vi "Knob Turn.vi"(0 "GEA2 Reference In":refnum<k24>, 7 "Button":T1=enum."Position 1", 11 "Error In":errorcluster) -> (4 "GEA2 Reference Out":refnum<k24>, 15 "Error Out":errorcluster)   [LabVIEW 2018, in "TL27.lvlib"]
uses:
  Projects/TL27.lvlib
  type defs/Encoder Position.ctl
  D:/Common/LabVIEW GEA2 Toolkit/source/GEA3 DLL Source/GeaCommunication.dll
  Common/LabVIEW GEA2 Toolkit/source/GEA3 DLL Source/GeaCommunication.dll
  Common/LabVIEW GEA2 Toolkit/GEA3/type defs/Source_Destination.ctl
  Common/LabVIEW GEA2 Toolkit/GEA3/type defs/ERD Write Data In.ctl
  Common/LabVIEW GEA2 Toolkit/GEA3/type defs/Data Type.ctl
  C:/Users/iallatyp/Desktop/New folder/GEA3/library/GEA2_Toolkit.lvlib
panel:
  in  "Standalone?":bool
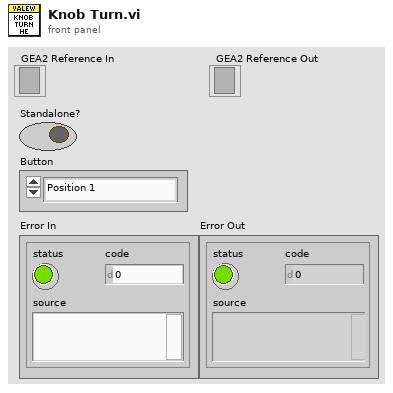
[diagram p1: front panel]
types:
  T1 = typedef "TL27.lvlib/Encoder Position.ctl" = enum16{"Position 0", "Position 1", "Position 2", "Position 3", "Position 4", "Position 5", "Position 6", "Position 7", "Position 8", "Position 9", "Position 10", "Position 11", "Position 12", "Position 13", "Clear / Reset"}
  T2 = typedef "GEA2_Toolkit.lvlib/ERD Write Data In.ctl" = cluster{"ERD Number":u16, "Data Type":T3, "Data":string}
  T3 = typedef "GEA2_Toolkit.lvlib/Data Type.ctl" = enum16{"string", "boolean", "uint8_t", "uint16_t", "uint32_t", "uint64_t", "int8_t", "int16_t", "int32_t", "int64_t"}
  T4 = typedef "GEA2_Toolkit.lvlib/Source_Destination.ctl" = cluster{"Source":u8, "Destination":u8}
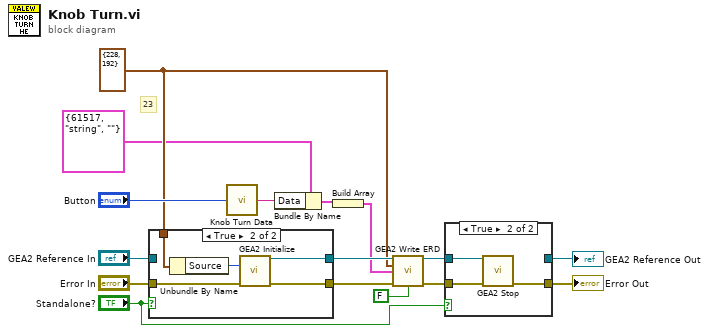
[diagram p0: block diagram]
diagram:
  w4 = T4 {"Source"=228, "Destination"=192} ("GEA Inputs")
  # "23"
  n1 = case shown="True" "Standalone?" {
    tunnel: "Error In" -> [w17 w23]
    tunnel: [w17 w22] -> w10
    tunnel: "GEA2 Reference In" -> [w18 _]
    tunnel: [w18 w21] -> w8
    tunnel: w4 -> [_ w19]
    frame False {
    }
    frame True {
      n2 = Unbundle By Name(w19) -> ("Source"=w20:u8)
      n3 = call "GEA2 Initialize.vi"("Source Address"=w20, "error in"=w23) -> ("GEA2 Reference Out"=w21:refnum<k24>, "error out"=w22:errorcluster)  [unwired: 11 in, 1 out]
    }
  }
  n4 = call "Knob Turn Data.vi"("Switch"="Button") -> ("Switch Message"=w7:string)  [unwired: 14 in]
  n5 = Bundle By Name(cluster=T2 {"ERD Number"=61517, "Data Type"=enum."string", "Data"=""} ("ERD Write Data In"), "Data"=w7) -> (w6:T2)
  n6 = Build Array(w6) -> (w5:T2[])
  n7 = call "GEA2 Write ERD.vi"("GEA2 Reference In"=w8, "GEA Inputs"=w4, "Write ERD List"=w5, "Error In"=w10, "Verify ERD Response?"=FALSE) -> ("GEA2 Reference Out"=w3:refnum<k24>, "Error Out"=w9:errorcluster)  [unwired: 8 in, 1 out]
  n8 = case shown="True" "Standalone?" {
    tunnel: [w24 w28] -> w13
    tunnel: w3 -> [w25 w27]
    tunnel: [w25 _] -> w12
    tunnel: w9 -> [w24 w26]
    frame False {
    }
    frame True {
      n9 = call "GEA2 Stop.vi"("GEA2 Reference In"=w27, "Error In"=w26) -> ("Error Out"=w28:errorcluster)  [unwired: 13 in]
    }
  }
  "Error Out" <- w13
  "GEA2 Reference Out" <- w12
